vi "releaseSlaving.vi"(8 "error in (no error)":errorcluster, 11 "Tapedrive_ESP301 in":refnum<class "Tapedrive_ESP301.lvclass">) -> (0 "error out":errorcluster, 3 "Tapedrive_ESP301 out":refnum<class "Tapedrive_ESP301.lvclass">)   [LabVIEW 2013, in "Tapedrive_ESP301.lvclass"]
uses:
  Tapedrive_ESP301.lvclass
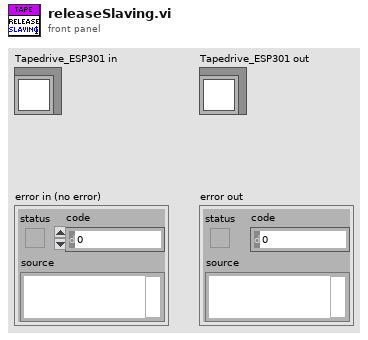
[diagram p1: front panel]
types:
  T1 = enum16{"Trapezoidal Mode", "S-curve Mode", "Jog Mode", "Slave to master's desired position (trajectory)", "Slave to master's actual position (feedback)", "Slave to master's actual velocity for jogging"}
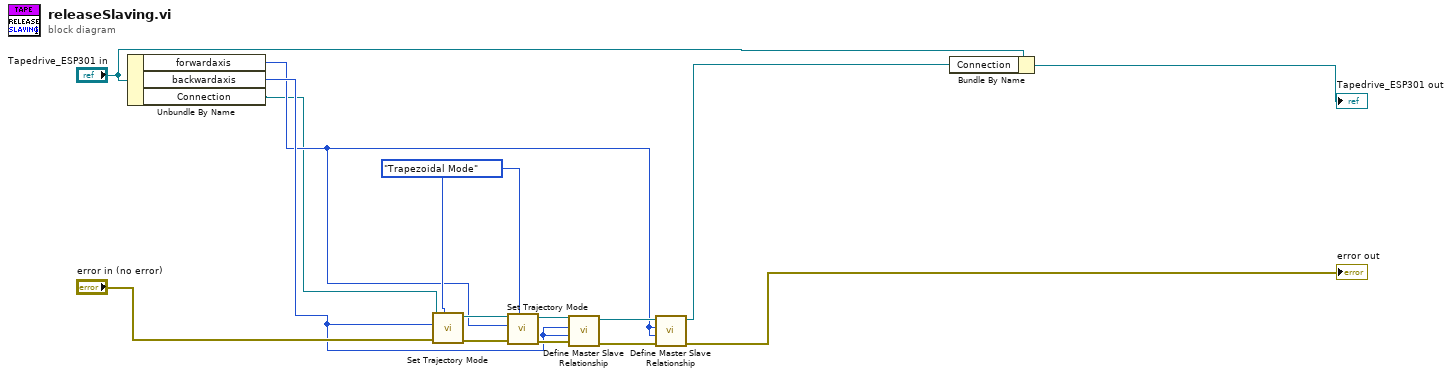
[diagram p0: block diagram]
diagram:
  w11 = T1."Trapezoidal Mode" ("Trajectory Mode")
  n1 = Unbundle By Name("Tapedrive_ESP301 in") -> ("forwardaxis"=w3:i16, "backwardaxis"=w4:i16, "Connection"=w1:refnum<visa-resource-name>)
  n2 = call <instrlib>:"Set Trajectory Mode.vi"("Trajectory Mode"=w11, "error in (no error)"="error in (no error)", "Axis (1)"=w4, "VISA resource name"=w1) -> ("error out"=w9:errorcluster, "VISA resource name out"=w10:refnum<visa-resource-name>)  [unwired: 3 in]
  n3 = call <instrlib>:"Set Trajectory Mode.vi"("Trajectory Mode"=w11, "error in (no error)"=w9, "Axis (1)"=w3, "VISA resource name"=w10) -> ("error out"=w15:errorcluster, "VISA resource name out"=w14:refnum<visa-resource-name>)  [unwired: 3 in]
  n4 = call <instrlib>:"Define Master Slave Relationship.vi"("error in (no error)"=w15, "Master Axis"=w4, "Slave Axis"=w4, "VISA resource name"=w14) -> ("error out"=w12:errorcluster, "VISA resource name out"=w13:refnum<visa-resource-name>)  [unwired: 2 in]
  n5 = call <instrlib>:"Define Master Slave Relationship.vi"("error in (no error)"=w12, "Master Axis"=w3, "Slave Axis"=w3, "VISA resource name"=w13) -> ("error out"=→"error out":errorcluster, "VISA resource name out"=w2:refnum<visa-resource-name>)  [unwired: 2 in]
  n6 = Bundle By Name(cluster="Tapedrive_ESP301 in", "Connection"=w2) -> (→"Tapedrive_ESP301 out":refnum<class "Tapedrive_ESP301.lvclass">)
